vi "PID Preference.vi"(0 "key":string, 1 "section":string, 2 "Operation":enum16{"Load", "Save"}(ring)=enum."Save", 3 "refnum in":T2, 9 "default value":T1={"high"=1.0, "low"=-1.0, "P"=1.0, "I"=0.0, "D"=0.0}) -> (12 "section out":string, 13 "Operation out":enum16{"Load", "Save"}(ring)=enum."Save", 14 "refnum out":T2)   [LabVIEW 2013]
uses:
  <vilib>/Utility/config.llb/Config Data RefNum.ctl
  Double Preference.vi
  <vilib>/Rock Robotics/Network Tables/SD Write Number.vi
  <vilib>/Utility/config.llb/Read Key.vi
  <vilib>/Utility/config.llb/Read Key (Double).vi
  <vilib>/Utility/config.llb/Write Key.vi
  <vilib>/Utility/config.llb/Write Key (Double).vi
  <vilib>/Rock Robotics/Network Tables/SD Read Number.vi
  <vilib>/Utility/config.llb/NI_LVConfig.lvlib
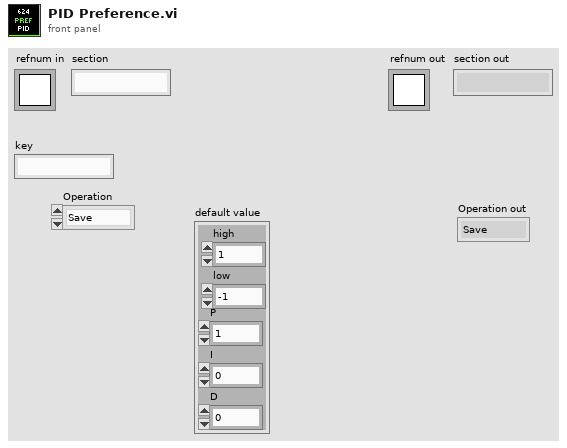
[diagram p1: front panel]
types:
  T1 = cluster{"high":dbl, "low":dbl, "P":dbl, "I":dbl, "D":dbl}
  T2 = typedef "NI_LVConfig.lvlib/Config Data RefNum.ctl" = refnum<k1>
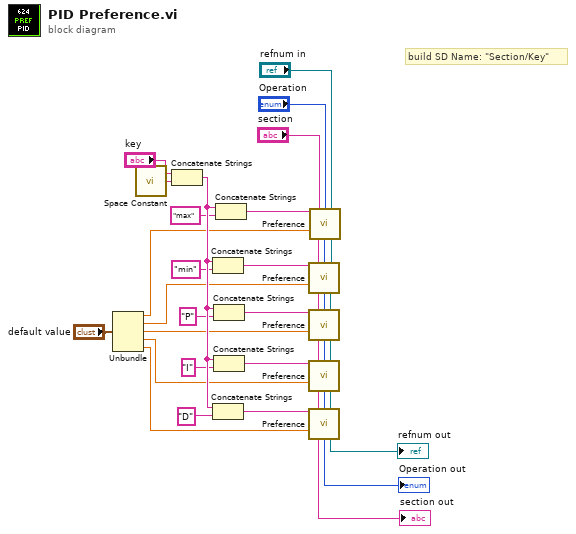
[diagram p0: block diagram]
diagram:
  # "build SD Name: \"Section/Key\""
  n1 = Unbundle("default value") -> ("high"=w1:dbl, "low"=w2:dbl, "P"=w3:dbl, "I"=w4:dbl, "D"=w5:dbl)
  n2 = call <vilib>:"Space Constant.vi"() -> ("String"=w36:string)
  n3 = Concatenate Strings("key", w36) -> (w37:string)
  n4 = Concatenate Strings(w37, "min" ("Name")) -> (w13:string)
  n5 = Concatenate Strings(w37, "D" ("Name")) -> (w10:string)
  n6 = Concatenate Strings(w37, "P" ("Name")) -> (w12:string)
  n7 = Concatenate Strings(w37, "I" ("Name")) -> (w11:string)
  n8 = Concatenate Strings(w37, "max" ("Name")) -> (w14:string)
  n9 = call-poly "Preference.vi"("key"=w14, "section"="section", "Operation"="Operation", "refnum in"="refnum in", "default value"=w1) -> ("section out"=w27:string, "Operation out"=w29:enum16{"Load", "Save"}, "refnum out"=w28:T2)  [unwired: 8 in]
  n10 = call-poly "Preference.vi"("key"=w13, "section"=w27, "Operation"=w29, "refnum in"=w28, "default value"=w2) -> ("section out"=w23:string, "Operation out"=w22:enum16{"Load", "Save"}, "refnum out"=w21:T2)  [unwired: 8 in]
  n11 = call-poly "Preference.vi"("key"=w12, "section"=w23, "Operation"=w22, "refnum in"=w21, "default value"=w3) -> ("section out"=w19:string, "Operation out"=w20:enum16{"Load", "Save"}, "refnum out"=w18:T2)  [unwired: 8 in]
  n12 = call-poly "Preference.vi"("key"=w11, "section"=w19, "Operation"=w20, "refnum in"=w18, "default value"=w4) -> ("section out"=w17:string, "Operation out"=w16:enum16{"Load", "Save"}, "refnum out"=w15:T2)  [unwired: 8 in]
  n13 = call-poly "Preference.vi"("key"=w10, "section"=w17, "Operation"=w16, "refnum in"=w15, "default value"=w5) -> ("section out"=→"section out":string, "Operation out"=→"Operation out":enum16{"Load", "Save"}, "refnum out"=→"refnum out":T2)  [unwired: 8 in]
